vi "Measure.vi"(8 "error in":errorcluster, 10 "Measure Type":i32(ring) items=["Current", "Power", "Voltage", "Capacity"], 11 "VISA resource name":refnum<visa-resource-name>) -> (0 "error out":errorcluster, 1 "返回数":u32, 2 "Value":dbl, 3 "VISA resource name out":refnum<visa-resource-name>)   [LabVIEW 2018, in "IT-M3100.lvlib"]
doc: "The command to get the following average.\n\n<b>Measure Type</b>\n0:Current:Return the current average of measurements.\n1:Power:Return to measure the power of the average.\n2:Voltage:Average return to measure the voltage.\n3:Capacity:Returns the capacity of battery charging and discharging."
uses:
  IT-M3100.lvlib
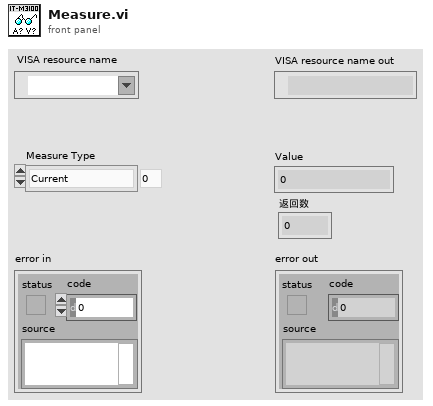
[diagram p1: front panel]
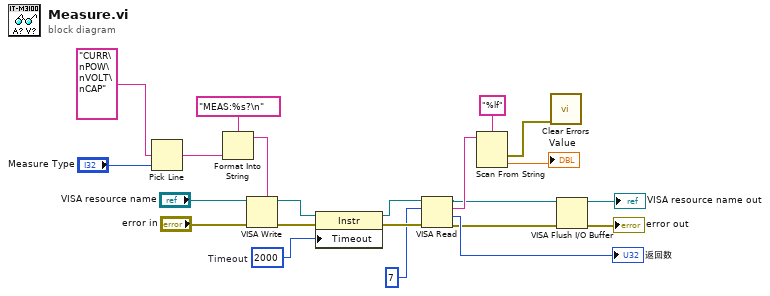
[diagram p0: block diagram]
diagram:
  w6 = u32 2000  # Timeout
  n1 = Pick Line(multi-line string="CURR\nPOW\nVOLT\nCAP", line index="Measure Type") -> (output string=w16:string)  [unwired: 1 in]
  n2 = Format Into String(format string="MEAS:%s?\n", w16) -> (resulting string=w19:string)  [unwired: 2 in, 1 out]
  n3 = VISA Write(VISA resource name="VISA resource name", write buffer=w19, error in (no error)="error in") -> (VISA resource name out=w7:refnum<visa-resource-name>, error out=w11:errorcluster)  [unwired: 1 out]
  n4 = property class="Instr"(reference=w7, error in=w11, "Timeout"=w6) -> (reference out=w10:refnum<visa-resource-name>, error out=w9:errorcluster)
  n5 = VISA Read(VISA resource name=w10, byte count=7, error in (no error)=w9) -> (VISA resource name out=w2:refnum<visa-resource-name>, read buffer=w21:string, return count=→"返回数":u32, error out=w1:errorcluster)
  n6 = Scan From String(format string="%lf", input string=w21) -> (error out=w8:errorcluster, output 1=→"Value":dbl)  [unwired: 3 in, 2 out]
  n7 = call <vilib>:"Clear Errors.vi"("error in (no error)"=w8) -> ()  [unwired: 5 in, 2 out]
  n8 = VISA Flush I/O Buffer(VISA resource name=w2, error in (no error)=w1) -> (VISA resource name out=→"VISA resource name out":refnum<visa-resource-name>, error out=→"error out":errorcluster)  [unwired: 1 in]
